vi "Check.vi"() -> ()   [LabVIEW 2019]
uses:
  Z_OnSwitch.xctl
  Y_source.ctl
  Z_State.ctl
  Logik/Logik.lvlib
  Heating.lvlib
panel:
  in  "Z_State_heating":T1=enum."on"
  out "Boolean":bool
  in  "Z_Source":T2
  in  "connect":bool
  in  "Z_OnSwitch":bool(xcontrol)
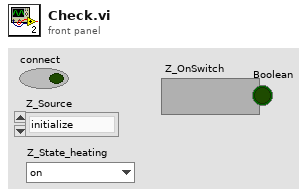
[diagram p1: front panel]
types:
  T1 = typedef "Heating.lvlib/Z_State.ctl" = enum8{"initialization", "alarm", "disabled", "not ready", "stop ready", "reserv", "switched off", "reserv2", "switched on", "check", "on min", "decrease out", "on", "increase out", "on max"}
  T2 = typedef "Heating.lvlib/Y_source.ctl" = enum8{"initialize", "local disabled", "local hand", "hand", "auto", "dist"}
  T3 = cluster{"connect":bool, "Z_Source":T2, "Z_State_heating":T1}
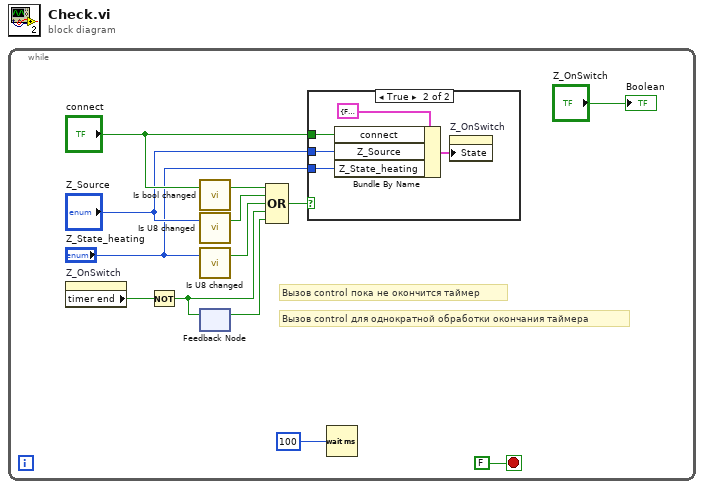
[diagram p0: block diagram]
diagram:
  n1 = while {
    stop <- FALSE stop-if-true
    # "Вызов control пока не окончится таймер"
    # "Вызов control для однократной обработки окончания таймера"
    n2 = property on="Z_OnSwitch" class="Z_OnSwitch (strict)"() -> ("timer end"=w5:bool)  [unwired: 2 in, 2 out]
    n3 = Not(x=w5) -> (.not. x?=w2:bool)
    n4 = call "Is bool changed.vi"("in"="connect") -> ("changed or first call?"=w8:bool)  [unwired: 2 in]
    n5 = call "Is U8 changed.vi"("in"="Z_Source") -> ("changed or first call?"=w9:bool)  [unwired: 2 in]
    n6 = call "Is U8 changed.vi"("in"="Z_State_heating") -> ("changed or first call?"=w1:bool)  [unwired: 2 in]
    n7 = feedback #1() -> (w3:bool)  [unwired: 1 in]
    n8 = feedback-in #1(w2) -> ()
    n9 = Compound Arithmetic op=OR(w8, w9, w1, w2, w3) -> (w11:bool)
    n10 = case shown="True" w11 {
      tunnel: "connect" -> [_ w18]
      tunnel: "Z_Source" -> [_ w17]
      tunnel: "Z_State_heating" -> [_ w16]
      frame False {
      }
      frame True {
        n11 = Bundle By Name(cluster=T3 {"connect"=FALSE, "Z_Source"=enum."initialize", "Z_State_heating"=enum."initialization"} ("source"), "connect"=w18, "Z_Source"=w17, "Z_State_heating"=w16) -> (w14:T3)
        n12 = property on="Z_OnSwitch" class="Z_OnSwitch (strict)"("State"=w14) -> ()  [unwired: 2 in, 2 out]
      }
    }
    n13 = Wait (ms)(milliseconds to wait=u32 100) -> ()  [unwired: 1 out]
    "Boolean" <- "Z_OnSwitch"
  }
